vi "FABR-Plot Traces.vi"(0 "Analysis":T1, 2 "Neural Ref":refnum<vi>, 9 "Normalize individual?":bool, 11 "error in (no error)":errorcluster, 12 "Scale":dbl) -> (15 "error out":errorcluster)   [LabVIEW 2020]
uses:
  Typedefs/FABR-Analysis State.ctl
  Threshold Estimation VIs/ABR3-Threshold Estimation Result.ctl
  epl-vi-lib/Utility VIs/Math VIs/LinSpace (x0-dx-npts).vi
panel:
  # "Freq X Level X Time"
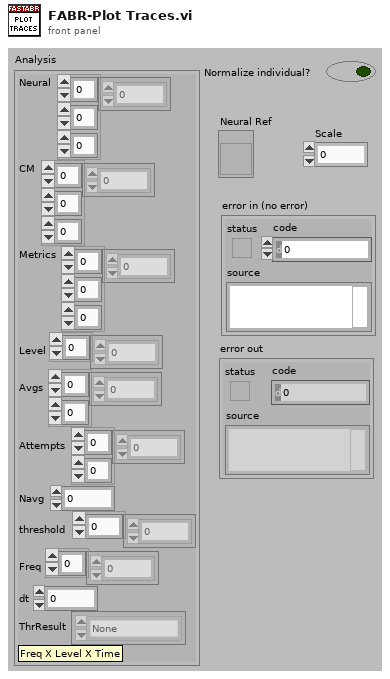
[diagram p1: front panel]
types:
  T1 = typedef "FABR-Analysis State.ctl" = cluster{"Neural":dbl[][][], "CM":dbl[][][], "Metrics":dbl[][][], "Level":dbl[], "Avgs":i32[][], "Attempts":i32[][], "Navg":i32, "threshold":dbl[], "Freq":dbl[], "dt":dbl, "ThrResult":T2[]}
  T2 = typedef "ABR3-Threshold Estimation Result.ctl" = enum16{"None", "Power", "Sigmoid", "Power (noisy)", "Suprathreshold", "Invalid"}
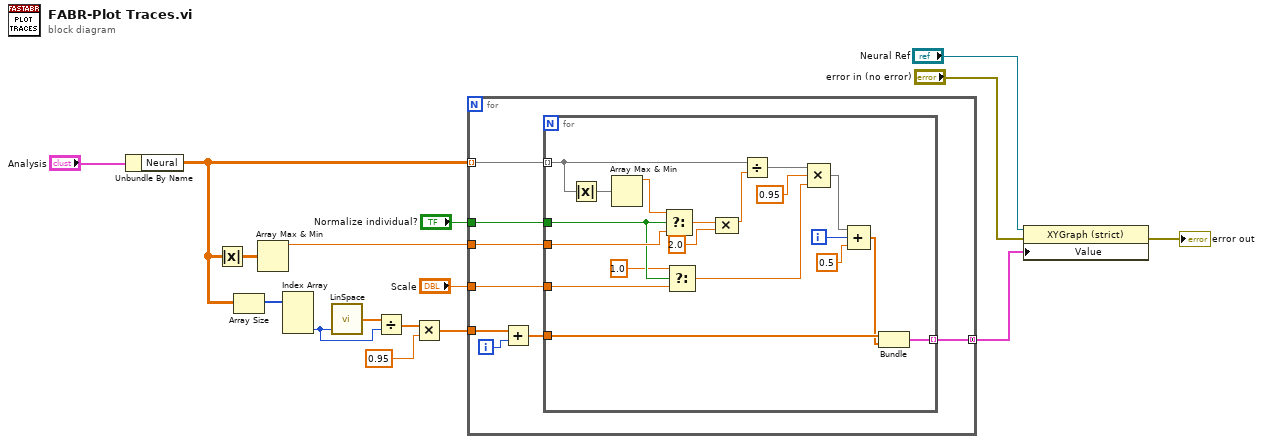
[diagram p0: block diagram]
diagram:
  n1 = Unbundle By Name("Analysis") -> ("Neural"=w15:dbl[][][])
  n2 = Absolute Value(x=w15) -> (abs(x)=w5:dbl[][][])
  n3 = Array Size(array=w15) -> (size(s)=w14:i32[])
  n4 = Array Max & Min(array=w5) -> (max value=w8:dbl)  [unwired: 3 out]
  n5 = Index Array(array=w14) -> (element #3=w12:i32)  [unwired: 3 in, 2 out]
  n6 = call-poly "LinSpace.vi"("npts"=w12) -> ("Array"=w13:dbl[])  [unwired: 3 in, 1 out]
  n7 = Divide(x=w13, y=w12) -> (x/y=w11:dbl[])
  n8 = Multiply(x=w11, y=0.95) -> (x*y=w9:dbl[])
  n9 = for {
    tunnel: w15 -> [w24] mode=indexing
    tunnel: w9 -> [w23]
    tunnel: w8 -> [w20]
    tunnel: [w19] -> w6 mode=concatenating
    tunnel: "Normalize individual?" -> [w18]
    tunnel: "Scale" -> [w17]
    i -> [w21]
    n10 = Add(x=w23, y=w21) -> (x+y=w22:dbl[])
    n11 = for {
      tunnel: w24 -> [w31] mode=indexing
      tunnel: w22 -> [w41]
      tunnel: w20 -> [w35]
      tunnel: [w39] -> w19 mode=indexing
      tunnel: w18 -> [w28]
      tunnel: w17 -> [w27]
      i -> [w37]
      n12 = Absolute Value(x=w31) -> (abs(x)=w32:dbl[])
      n13 = Array Max & Min(array=w32) -> (max value=w30:dbl)  [unwired: 3 out]
      n14 = Select(t=w30, s=w28, f=w35) -> (s? t:f=w34:dbl)
      n15 = Select(t=1.0, s=w28, f=w27) -> (s? t:f=w25:dbl)
      n16 = Compound Arithmetic op=MULTIPLY(w34, 2.0 ("y")) -> (w33:dbl)
      n17 = Divide(x=w31, y=w33) -> (x/y=w43:dbl[])
      n18 = Compound Arithmetic op=MULTIPLY(w43, 0.95, w25) -> (w40:dbl[])
      n19 = Compound Arithmetic op=unknown(w40, w37, 0.5) -> (w38:dbl[])
      n20 = Bundle(w41, w38) -> (w39:cluster{dbl[], dbl[]})  [unwired: 1 in]
    }
  }
  n21 = property class="XYGraph (strict)"(reference="Neural Ref", error in="error in (no error)", "Value"=w6) -> (error out=→"error out":errorcluster)  [unwired: 1 out]
